vi "main.vi"   [LabVIEW 2017]
uses:
  DAQ/DAQ.lvlib
  DAQ/DAQ.Global.vi
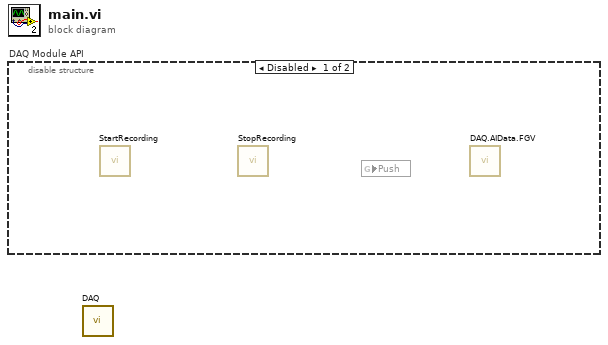
[diagram p0: block diagram]
diagram:
  n1 = disable-structure "DAQ Module API" shown="Disabled" {
    frame Disabled {
      n2 = call "StartRecording.vi"() -> ()  [unwired: 11 in, 1 out]
      n3 = call "StopRecording.vi"() -> ()  [unwired: 11 in, 1 out]
      n4 = global read "DAQ.Global.vi" "Push"() -> ()  [unwired: 1 in]
      n5 = call "DAQ.AIData.FGV.vi"() -> ()  [unwired: 10 in, 2 out]
    }
    frame Enabled {
    }
  }
  n6 = call "DAQ.vi"() -> ()  [unwired: 12 in]
